vi "CustomerDeviceSelect.vi"() -> ()   [LabVIEW 2012]
uses:
  <vilib>/addons/database/Auxilliary.llb/DB Tools Cursor Type.ctl
  <vilib>/addons/database/Connection.llb/DB Tools Open Connec (Path).vi
  <vilib>/addons/database/Connection.llb/Conn Execute.vi
  <vilib>/addons/database/Recordset.llb/Rec Fetch Recordset Data (R).vi
  <vilib>/addons/database/Recordset.llb/Rec Destroy - Connection.vi
  <vilib>/addons/database/_DB Variant To Data/Database Variant To Data.xnode
  <vilib>/addons/database/NI_Database_API.lvlib
panel:
  in  "Device":string(combo)
  in  "connection information":path=path "e:/m100/data/m1003.dsn"
  in  "input cluster":cluster{"String":string, "Value":string}
  out "error out":errorcluster
  in  "error in (no error)":errorcluster
  in  "Customer":string(combo)
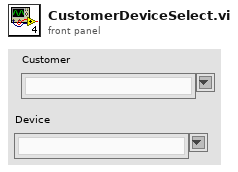
[diagram p1: front panel]
types:
  T1 = typedef "NI_Database_API.lvlib/DB Tools Cursor Type.ctl" = enum16{"forward-only", "keyset", "dynamic", "static"}
  T2 = typedef "NI_Database_API.lvlib/Conn ObjectReference.ctl" = refnum<k1>
  T3 = typedef "NI_Database_API.lvlib/Rec ObjectReference.ctl" = refnum<k1>
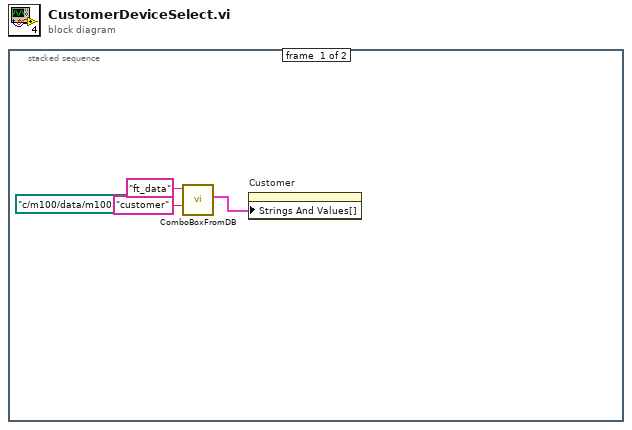
[diagram p0: block diagram]
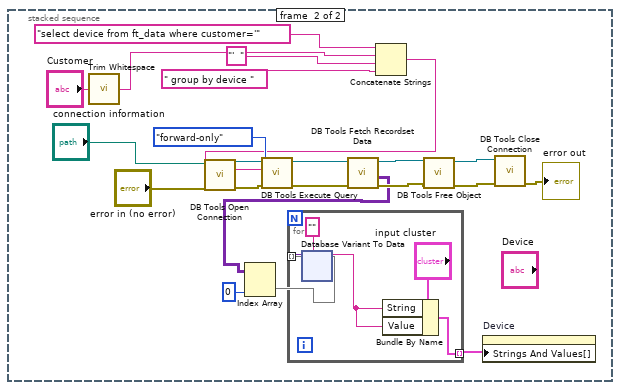
[diagram p2: hidden frame]
diagram:
  n1 = stacked-sequence {
    frame #0 {
      n2 = call "ComboBoxFromDB.vi"("connection information"=path "c:/m100/data/m1003.dsn", "Column"="customer", "table"="ft_data") -> ("Array"=w1:cluster{"String":string, "Value":string}[])  [unwired: 7 in, 1 out]
      n3 = property on="Customer" class="CmbBox"("Strings And Values[]"=w1) -> ()  [unwired: 2 in, 2 out]
    }
    frame #1 {
      n4 = call <vilib>:"Trim Whitespace.vi"("string"="Customer") -> ("trimmed string"=w5:string)  [unwired: 1 in]
      n5 = call-poly <vilib>:"DB Tools Open Connection.vi"("error in (no error)"="error in (no error)", "connection information"="connection information") -> ("error out"=w23:errorcluster, "connection reference"=w24:T2)  [unwired: 6 in]
      n6 = Concatenate Strings("select device from ft_data where customer='" ("string"), w5, "'  " ("string"), " group by device " ("string")) -> (w10:string)
      n7 = call-poly <vilib>:"DB Tools Execute Query.vi"("error in (no error)"=w23, "cursor type"=DB_Tools_Cursor_Type."forward-only", "SQL query"=w10, "connection reference"=w24) -> ("error out"=w18:errorcluster, "recordset reference"=w19:T3)  [unwired: 4 in]
      n8 = call-poly <vilib>:"DB Tools Fetch Recordset Data.vi"("error in (no error)"=w18, "recordset reference"=w19) -> ("error out"=w16:errorcluster, "recordset data"=w15:variant[][], "recordset reference out"=w17:T3)  [unwired: 3 in]
      n9 = Index Array(array=w15, index (col)=0) -> (element=w14:variant[])  [unwired: 1 in]
      n10 = for {
        tunnel: w14 -> [w31] mode=indexing
        tunnel: [w27] -> w7 mode=indexing
        n11 = xnode "Database Variant To Data"("database variant"=w31, "type"="") -> ("data"=w28:string)  [unwired: 1 in, 1 out]
        n12 = Bundle By Name(cluster="input cluster", "String"=w28, "Value"=w28) -> (w27:cluster{"String":string, "Value":string})
      }
      n13 = call-poly <vilib>:"DB Tools Free Object.vi"("error in (no error)"=w16, "recordset reference"=w17) -> ("error out"=w21:errorcluster, "connection reference"=w22:T2)  [unwired: 8 in]
      n14 = property on="Device" class="CmbBox"("Strings And Values[]"=w7) -> ()  [unwired: 2 in, 2 out]
      n15 = call <vilib>:"DB Tools Close Connection.vi"("error in (no error)"=w21, "connection reference"=w22) -> ("error out"=→"error out":errorcluster)  [unwired: 5 in]
    }
  }
